vi "AlazarFFTSetWindowFunction.vi"(0 "DSP Handle":u64, 5 "Samples per record":u32, 7 "Real window array":sgl[](array[numeric]), 9 "Imag window array":sgl[](array[numeric]), 11 "error in (no error)":errorcluster) -> (4 "DSP Handle":u64, 15 "error out":errorcluster)   [LabVIEW 2009]
uses:
  ATSApi.dll
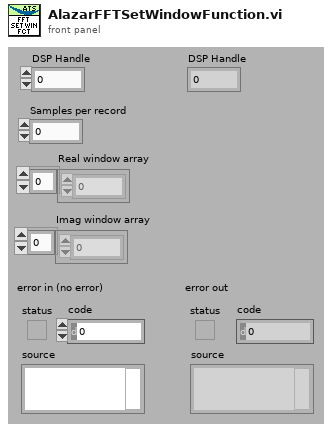
[diagram p1: front panel]
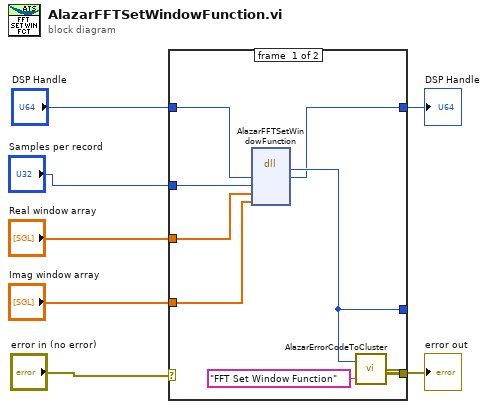
[diagram p0: block diagram]
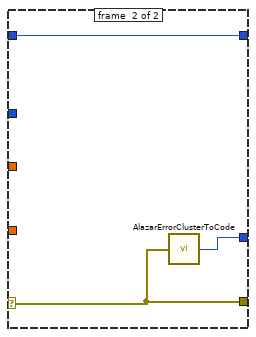
[diagram p2: hidden frame]
diagram:
  n1 = case shown="No Error" "error in (no error)" {
    selector: "error in (no error)" -> [_ w18]
    tunnel: [w12 w18] -> w6
    tunnel: [w14 w17] -> _
    tunnel: "DSP Handle" -> [w15 w16]
    tunnel: [w11 w16] -> w4
    tunnel: "Samples per record" -> [w10 _]
    tunnel: "Imag window array" -> [w9 _]
    tunnel: "Real window array" -> [w8 _]
    frame #0 {
      n2 = dll-call lib="ATSApi.dll" fn="AlazarFFTSetWindowFunction"("handle"=w15, "samplesPerRecord"=w10, "realWindowArray"=w8, "imagWindowArray"=w9) -> ("return type"=w14:u32, "handle"=w11:u64)  [unwired: 6 in, 2 out]
      n3 = call "AlazarErrorCodeToCluster.vi"("Message"="FFT Set Window Function", "Error Code"=w14) -> ("error out"=w12:errorcluster)
    }
    frame #1 {
      n4 = call "AlazarErrorClusterToCode.vi"("error in (no error)"=w18) -> ("Error Code"=w17:u32)
    }
  }
  "DSP Handle" <- w4
  "error out" <- w6
